vi "Knock Sensors Page.vi"(8 "error in (no error)":errorcluster, 11 "Node Ptr":T1 format="%.0x") -> (0 "error out":errorcluster)   [LabVIEW 2019, in "Engine Simulation Toolkit System Explorer.lvlib"]
uses:
  Engine Simulation Toolkit System Explorer.lvlib
  <vilib>/NI VeriStand/Custom Device API/Custom Device Item Ref.ctl
  Shared/Properties.vi
  Shared/Constants and GUIDs.vi
  <vilib>/NI VeriStand/Custom Device API/Custom Device API.lvlib
  Shared/Engine Simulation Toolkit Shared.lvlib
  <vilib>/NI VeriStand/Custom Device Tools/Custom Device Utility Library/Custom Device Utility Library.lvlib
panel:
  in  "remove":bool
  in  "add":bool
  in  "Knock listbox":i32[](listbox) caption="Available Knock Sensors"
  in  "Header":cluster{"Section Name":string}={"Section Name"="Knock Sensors"}
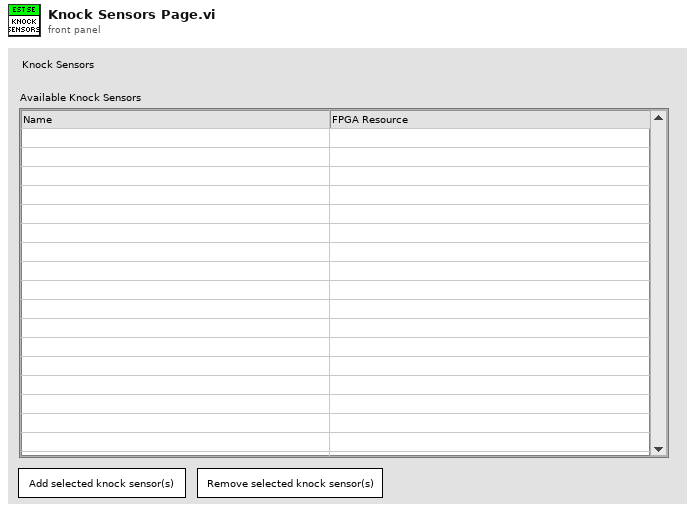
[diagram p1: front panel]
types:
  T1 = typedef "Custom Device API.lvlib/Custom Device Item Ref.ctl" = u64
  T2 = enum8{"Enabled", "Disabled", "Disabled and Grayed Out"}
  T3 = cluster{"ip list property name":string, string[]}[]
  T4 = typedef "Custom Device API.lvlib/Custom Device Commands.ctl" = enum16{"Default", "Item renamed", "Shutdown", "Dynamic button pressed"}
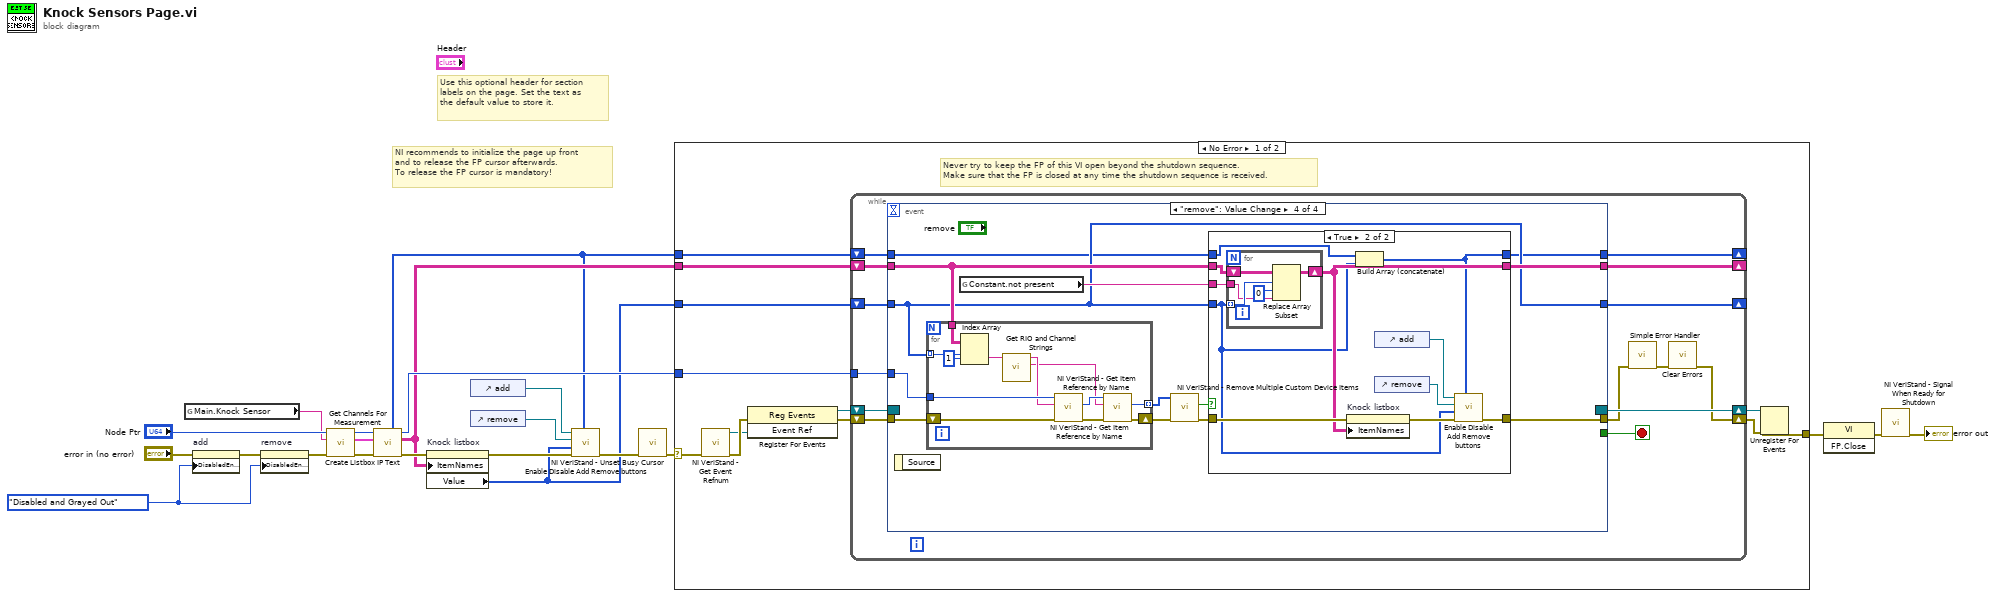
[diagram p0: block diagram]
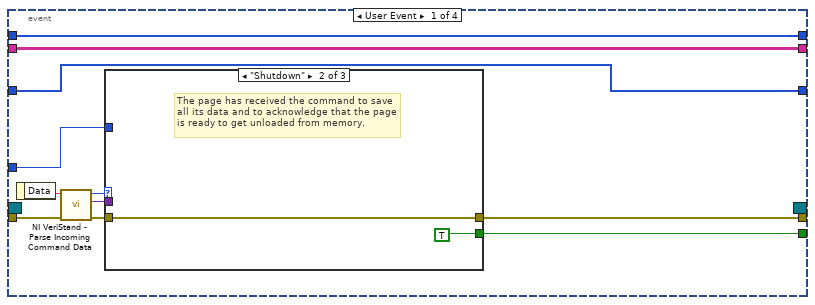
[diagram p2: hidden frame]
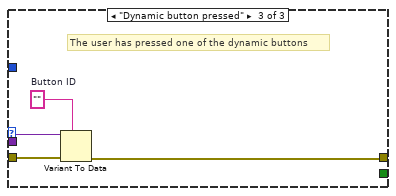
[diagram p4: hidden frame]
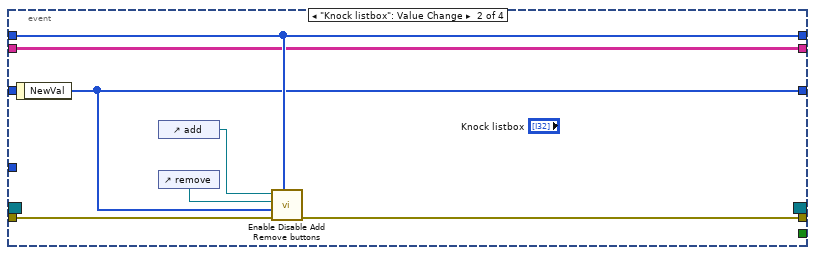
[diagram p5: hidden frame]
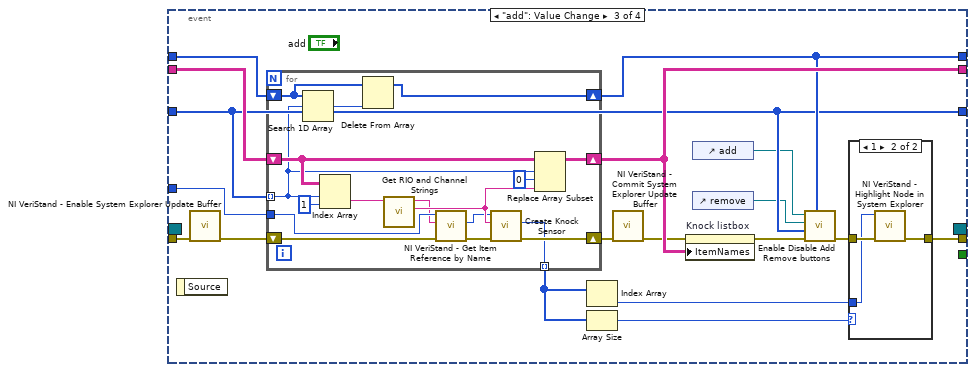
[diagram p6: hidden frame]
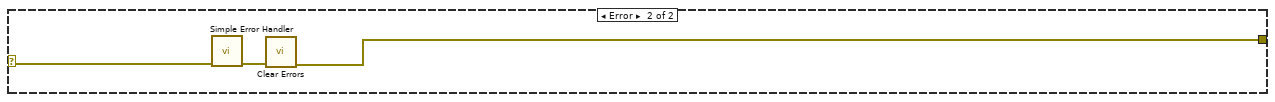
[diagram p9: hidden frame]
diagram:
  w13 = T2."Disabled and Grayed Out" ("Disabled")
  # "Use this optional header for section labels on the page. Set the text as the default value to store it."
  # "NI recommends to initialize the page up front\nand to release the FP cursor afterwards.\nTo release the FP cursor is mandatory!"
  n1 = global read "Properties.vi" "Main.Knock Sensor"() -> (w1:string)
  n2 = property on="add" class="Bool"(error in="error in (no error)", "DisabledEnum"=w13) -> (error out=w14:errorcluster)  [unwired: 1 in, 1 out]
  n3 = property on="remove" class="Bool"(error in=w14, "DisabledEnum"=w13) -> (error out=w3:errorcluster)  [unwired: 1 in, 1 out]
  n4 = call "Get Channels For Measurement.vi"("error in (no error)"=w3, "property name"=w1, "Node Ptr in"="Node Ptr") -> ("error out"=w6:errorcluster, "rios and channels"=w5:T3, "Node Ptr out"=w4:T1)  [unwired: 6 in]
  n5 = call "Create Listbox IP Text.vi"("error in (no error)"=w6, "rios and analog replays"=w5, "Section Ref in"=w4) -> ("error out"=w16:errorcluster, "listbox text"=w15:string[][], "Section Ref out"=w17:T1, "not present item indexes"=w8:i32[])  [unwired: 5 in]
  n6 = property on="Knock listbox" class="MCListbox (strict)"(error in=w16, "ItemNames"=w15) -> (error out=w10:errorcluster, "Value"=w7:i32[])  [unwired: 1 in, 1 out]
  n7 = control-ref of="add"() -> (w11:refnum<vi>)
  n8 = control-ref of="remove"() -> (w12:refnum<vi>)
  n9 = call "Enable Disable Add Remove buttons.vi"("not present item indexes"=w8, "error in (no error)"=w10, "selected items"=w7, "remove button"=w12, "add button"=w11) -> ("error out"=w9:errorcluster)  [unwired: 6 in]
  n10 = call <vilib>:"NI VeriStand - Unset Busy Cursor.vi"("error in (no error)"=w9) -> ("error out"=w19:errorcluster)  [unwired: 10 out]
  n11 = case shown="No Error" w19 {
    selector: w19 -> [w26 w159]
    tunnel: [w31 w157] -> w22
    tunnel: w17 -> [w27 _]
    tunnel: w15 -> [w25 _]
    tunnel: w8 -> [w24 _]
    tunnel: w7 -> [w23 _]
    frame No Error {
      # "Never try to keep the FP of this VI open beyond the shutdown sequence.\nMake sure that the FP is closed at any time the shutdown sequence is received."
      n12 = call <vilib>:"NI VeriStand - Get Event Refnum.vi"("error in (no error)"=w26) -> ("error out"=w34:errorcluster, "Event Ref"=w30:refnum<user-event>)  [unwired: 9 out]
      n13 = register-events(error in=w34, w30) -> (reference out=w28:refnum<event-registration>, error out=w29:errorcluster)  [unwired: 1 in]
      n14 = while {
        tunnel: w27 -> [w44]
        shift-right: [w41] -> w32
        shift-left: w29 -> [w47]
        shift-right: [w48] -> w33
        shift-left: w28 -> [w46]
        shift-right: [w38] -> _
        shift-left: w23 -> [w37]
        shift-right: [w35] -> _
        shift-left: w24 -> [w39]
        shift-right: [w36] -> _
        shift-left: w25 -> [w40]
        stop <- w45 stop-if-true
        n15 = event shown="[3] \"remove\": Value Change" {
          selector: w46 -> [_ _ _ _]
          dyn-events: [_ _ _ _] -> w48
          timeout: _ -> [_ _ _ _]
          tunnel: w47 -> [w59 w73 w91 w124]
          tunnel: [w55 _ _ _] -> w45
          tunnel: [w54 w72 w76 w125] -> w43
          tunnel: w44 -> [w53 _ w90 w123]
          tunnel: w40 -> [w50 w67 w89 w118]
          tunnel: w39 -> [w49 w69 w88 w114]
          tunnel: [w51 w68 w83 w115] -> w38
          tunnel: w37 -> [w51 _ w83 w115]
          tunnel: [w50 w67 w86 w116] -> w36
          tunnel: [w49 w69 w84 w113] -> w35
          event User Event {
            n16 = event-data() -> ("Data"=w58:string)  [unwired: 1 out]
            n17 = call <vilib>:"NI VeriStand - Parse Incoming Command Data.vi"("error in (no error)"=w59, "Incoming data"=w58) -> ("error out"=w57:errorcluster, "Outgoing data"=w52:variant, "Action"=w56:T4)  [unwired: 7 out]
            n18 = case shown="\"Shutdown\"" w56 {
              tunnel: w57 -> [w60 w61 w66]
              tunnel: [_ TRUE _] -> w55
              tunnel: [w60 w61 w63] -> w54
              tunnel: w53 -> [_ _ _]
              tunnel: w52 -> [_ _ w65]
              frame "Default", Default {
              }
              frame "Shutdown" {
                # "The page has received the command to save all its data and to acknowledge that the page is ready to get unloaded from memory."
              }
              frame "Dynamic button pressed" {
                w64 = ""  # Button ID
                # "The user has pressed one of the dynamic buttons"
                n19 = Variant To Data(error in=w66, type=w64, Variant=w65) -> (error out=w63:errorcluster)  [unwired: 1 out]
              }
            }
          }
          event "Knock listbox": Value Change {
            n20 = event-data() -> ("NewVal"=w68:i32[])  [unwired: 1 out]
            n21 = control-ref of="add"() -> (w71:refnum<vi>)
            n22 = control-ref of="remove"() -> (w70:refnum<vi>)
            n23 = call "Enable Disable Add Remove buttons.vi"("not present item indexes"=w69, "error in (no error)"=w73, "selected items"=w68, "remove button"=w70, "add button"=w71) -> ("error out"=w72:errorcluster)  [unwired: 6 in]
          }
          event "add": Value Change {
            n24 = event-data() -> ()  [unwired: 2 out]
            n25 = call <vilib>:"NI VeriStand - Enable System Explorer Update Buffer.vi"("error in (no error)"=w91) -> ("error out"=w79:errorcluster)  [unwired: 10 in]
            n26 = for {
              tunnel: w90 -> [w100]
              shift-right: [w112] -> w87
              shift-left: w79 -> [w96]
              tunnel: w83 -> [w107] mode=indexing
              shift-right: [w109] -> w86
              shift-left: w89 -> [w110]
              shift-right: [w104] -> w84
              shift-left: w88 -> [w106]
              tunnel: [w103] -> w78 mode=indexing
              n27 = Search 1D Array(1D array=w106, element=w107) -> (index of element=w105:i32)  [unwired: 1 in]
              n28 = Index Array(array=w110, index (row)=w107, index (col)=1 ("disabled index (col)")) -> (element=w102:string)
              n29 = Delete From Array(array=w106, index=w105) -> (array with subset deleted=w104:i32[])  [unwired: 1 in, 1 out]
              n30 = call "Get RIO and Channel Strings.vi"("rio/channel"=w102) -> ("channel"=w101:string, "rio"=w99:string)  [unwired: 9 in]
              n31 = call <vilib>:"NI VeriStand - Get Item Reference by Name.vi"("error in (no error)"=w96, "Item Name"=w99, "Parent Ref in"=w100) -> ("error out"=w97:errorcluster, "Item Ref"=w98:T1)  [unwired: 5 in, 2 out]
              n32 = call "Create Knock Sensor.vi"("error in (no error)"=w97, "knock sensor name"=w101, "Section Ptr"=w98) -> ("error out"=w112:errorcluster, "Knock sensor ref"=w103:T1)  [unwired: 6 in, 1 out]
              n33 = Replace Array Subset(array=w110, new element=w101, index (row)=w107, index (col)=0 ("disabled index (col)")) -> (w109:string[][])
            }
            n34 = Index Array(array=w78) -> (element=w74:T1)  [unwired: 1 in]
            n35 = Array Size(array=w78) -> (size(s)=w77:i32)
            n36 = call <vilib>:"NI VeriStand - Commit System Explorer Update Buffer.vi"("error in (no error)"=w87) -> ("error out"=w80:errorcluster)  [unwired: 10 in]
            n37 = property on="Knock listbox" class="MCListbox (strict)"(error in=w80, "ItemNames"=w86) -> (error out=w85:errorcluster)  [unwired: 1 in, 1 out]
            n38 = control-ref of="add"() -> (w82:refnum<vi>)
            n39 = control-ref of="remove"() -> (w81:refnum<vi>)
            n40 = call "Enable Disable Add Remove buttons.vi"("not present item indexes"=w84, "error in (no error)"=w85, "selected items"=w83, "remove button"=w81, "add button"=w82) -> ("error out"=w75:errorcluster)  [unwired: 6 in]
            n41 = case shown="1" w77 {
              tunnel: [w92 w94] -> w76
              tunnel: w75 -> [w92 w95]
              tunnel: w74 -> [_ w93]
              frame Default {
              }
              frame 1 {
                n42 = call <vilib>:"NI VeriStand - Highlight Node in System Explorer.vi"("error in (no error)"=w95, "Item Ref in"=w93) -> ("error out"=w94:errorcluster)  [unwired: 8 in, 1 out]
              }
            }
          }
          event "remove": Value Change {
            n43 = event-data() -> ()  [unwired: 2 out]
            n44 = for {
              tunnel: w115 -> [w155] mode=indexing
              tunnel: w118 -> [w156]
              tunnel: w123 -> [w152]
              tunnel: [w149] -> w121 mode=indexing
              shift-right: [w150] -> w122
              shift-left: w124 -> [w153]
              n45 = Index Array(array=w156, index (row)=w155, index (col)=1 ("disabled index (col)")) -> (element=w147:string)
              n46 = call "Get RIO and Channel Strings.vi"("rio/channel"=w147) -> ("channel"=w145:string, "rio"=w146:string)  [unwired: 9 in]
              n47 = call <vilib>:"NI VeriStand - Get Item Reference by Name.vi"("error in (no error)"=w153, "Item Name"=w146, "Parent Ref in"=w152) -> ("error out"=w151:errorcluster, "Item Ref"=w148:T1)  [unwired: 5 in, 2 out]
              n48 = call <vilib>:"NI VeriStand - Get Item Reference by Name.vi"("error in (no error)"=w151, "Item Name"=w145, "Parent Ref in"=w148) -> ("error out"=w150:errorcluster, "Item Ref"=w149:T1)  [unwired: 5 in, 2 out]
            }
            n49 = global read "Constants and GUIDs.vi" "Constant.not present"() -> (w117:string)
            n50 = call <vilib>:"NI VeriStand - Remove Multiple Custom Device Items.vi"("error in (no error)"=w122, "Item Refs in"=w121) -> ("error out"=w120:errorcluster, "Deleted?"=w119:bool)  [unwired: 8 in]
            n51 = case shown="True" w119 {
              tunnel: [w127 w138] -> w125
              tunnel: w120 -> [w127 w135]
              tunnel: w115 -> [_ w130]
              tunnel: w118 -> [w128 w134]
              tunnel: w117 -> [_ w133]
              tunnel: [w128 w132] -> w116
              tunnel: w114 -> [w126 w131]
              tunnel: [w126 w129] -> w113
              frame False {
              }
              frame True {
                n52 = for {
                  tunnel: w130 -> [w142] mode=indexing
                  shift-right: [w143] -> w132
                  shift-left: w134 -> [w144]
                  tunnel: w133 -> [w140]
                  n53 = Replace Array Subset(array=w144, new element=w140, index (row)=w142, index (col)=0 ("disabled index (col)")) -> (w143:string[][])
                }
                n54 = property on="Knock listbox" class="MCListbox (strict)"(error in=w135, "ItemNames"=w132) -> (error out=w139:errorcluster)  [unwired: 1 in, 1 out]
                n55 = Build Array (concatenate)(w131, w130) -> (w129:i32[])
                n56 = control-ref of="add"() -> (w137:refnum<vi>)
                n57 = control-ref of="remove"() -> (w136:refnum<vi>)
                n58 = call "Enable Disable Add Remove buttons.vi"("not present item indexes"=w129, "error in (no error)"=w139, "selected items"=w130, "remove button"=w136, "add button"=w137) -> ("error out"=w138:errorcluster)  [unwired: 6 in]
              }
            }
          }
        }
        n59 = call <vilib>:"Simple Error Handler.vi"("error in (no error)"=w43) -> ("error out"=w42:errorcluster)  [unwired: 1 in, 7 out]
        n60 = call <vilib>:"Clear Errors.vi"("error in (no error)"=w42) -> ("error out"=w41:errorcluster)  [unwired: 1 in, 5 out]
      }
      n61 = Unregister For Events(event registration refnum=w33, error in=w32) -> (error out=w31:errorcluster)
    }
    frame Error {
      n62 = call <vilib>:"Simple Error Handler.vi"("error in (no error)"=w159) -> ("error out"=w158:errorcluster)  [unwired: 1 in, 7 out]
      n63 = call <vilib>:"Clear Errors.vi"("error in (no error)"=w158) -> ("error out"=w157:errorcluster)  [unwired: 1 in, 5 out]
    }
  }
  n64 = invoke class="VI" method="FP.Close"(error in=w22) -> (error out=w21:errorcluster)  [unwired: 2 in, 2 out]
  n65 = call <vilib>:"NI VeriStand - Signal When Ready for Shutdown.vi"("error in (no error)"=w21) -> ("error out"=→"error out":errorcluster)  [unwired: 10 out]
